vi "Write Config Data.vi"(0 "AI Channel":string, 1 "Sample Rate":dbl, 2 "Samples per Channel":i32, 3 "AO Channel":string, 5 "Error In":errorcluster) -> (14 "configuration file out":path, 19 "Error Out":errorcluster)   [LabVIEW 2020]
uses:
  <vilib>/Utility/config.llb/Write Key (String).vi
  <vilib>/Utility/config.llb/Write Key (Double).vi
  <vilib>/Utility/config.llb/Write Key (I32).vi
  <vilib>/Utility/config.llb/NI_LVConfig.lvlib
panel:
  # "Analog Input Channel Configuration"
  # "Analog Output Channel Configuration"
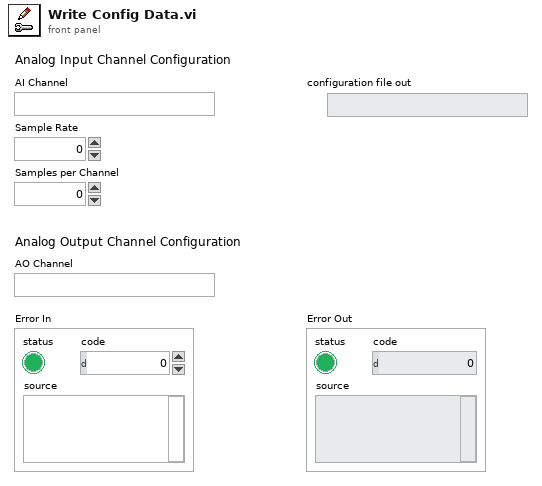
[diagram p1: front panel]
types:
  T1 = typedef "NI_LVConfig.lvlib/Config Data RefNum.ctl" = refnum<k1>
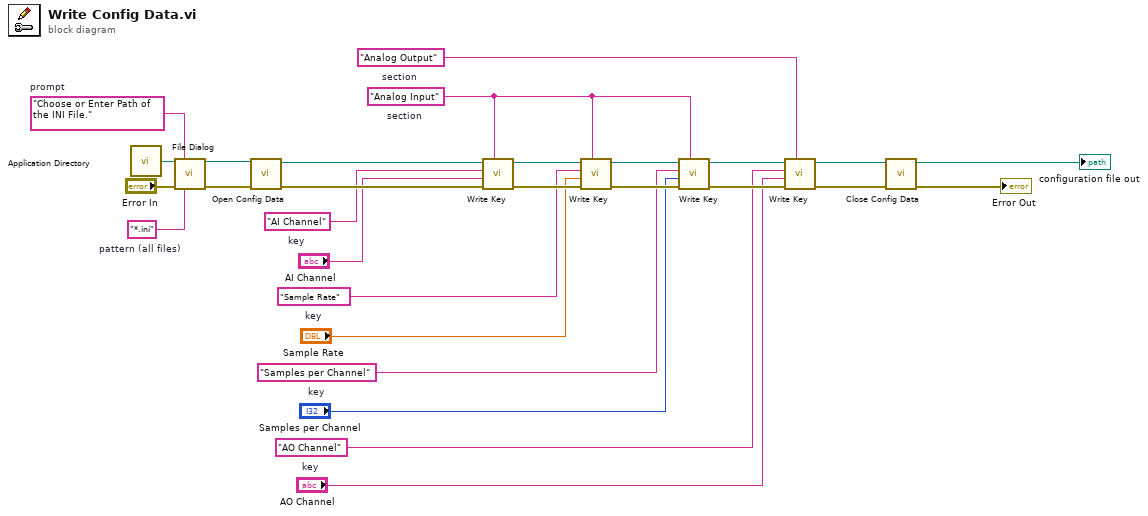
[diagram p0: block diagram]
diagram:
  w5 = "Analog Output"  # section
  w8 = "AO Channel"  # key
  w12 = "Samples per Channel"  # key
  w16 = "Sample Rate"  # key
  w6 = "Analog Input"  # section
  w20 = "AI Channel"  # key
  w25 = "*.ini"  # pattern (all files)
  w27 = "Choose or Enter Path of the INI File."  # prompt
  n1 = call <vilib>:"Application Directory.vi"() -> ("Application Directory"=w28:path)
  n2 = call "File Dialog"("start path"=w28, "prompt"=w27, "error in"="Error In", "pattern (all files)"=w25) -> ("selected path"=w23:path, "error out"=w24:errorcluster)  [unwired: 8 in, 2 out]
  n3 = call <vilib>:"Open Config Data.vi"("error in (no error)"=w24, "configuration file path"=w23) -> ("error out"=w21:errorcluster, "refnum"=w22:T1)  [unwired: 7 in, 1 out]
  n4 = call-poly <vilib>:"Write Key.vi"("section"=w6, "error in (no error)"=w21, "value"="AI Channel", "key"=w20, "refnum"=w22) -> ("error out"=w17:errorcluster, "refnum out"=w18:T1)  [unwired: 4 in, 1 out]
  n5 = call-poly <vilib>:"Write Key.vi"("section"=w6, "error in (no error)"=w17, "value"="Sample Rate", "key"=w16, "refnum"=w18) -> ("error out"=w13:errorcluster, "refnum out"=w14:T1)  [unwired: 4 in, 1 out]
  n6 = call-poly <vilib>:"Write Key.vi"("section"=w6, "error in (no error)"=w13, "value"="Samples per Channel", "key"=w12, "refnum"=w14) -> ("error out"=w9:errorcluster, "refnum out"=w10:T1)  [unwired: 4 in, 1 out]
  n7 = call-poly <vilib>:"Write Key.vi"("section"=w5, "error in (no error)"=w9, "value"="AO Channel", "key"=w8, "refnum"=w10) -> ("error out"=w4:errorcluster, "refnum out"=w3:T1)  [unwired: 4 in, 1 out]
  n8 = call <vilib>:"Close Config Data.vi"("error in (no error)"=w4, "refnum"=w3) -> ("error out"=→"Error Out":errorcluster, "file path"=→"configuration file out":path)  [unwired: 8 in]
